vi "read_lia.vi"(5 "Samples per step":i32, 6 "Reference Source (0: Internal)":i32(ring)=1 items=["Internal", "External", "Dual", "Chop"], 7 "error in (no error)":errorcluster, 8 "Single Lock-in Parameter 2 (0: X output)":i32(ring)=3 items=["X output", "Y output", "R output", "Theta output", "Aux In 1", "Aux In 2", "Aux In 3", "Aux In 4", "Aux Out 1", "Aux Out 2", "Xnoise", "Ynoise", "Reference Phase", "Sine Out Amplitude", "DC Level", "Int. Ref. Frequency", "Ext. Ref. Frequency"], 9 "Single Lock-in Parameter (0: X output)":u16(ring)=2 items=["X output", "Y output", "R output", "Theta output", "Aux In 1", "Aux In 2", "Aux In 3", "Aux In 4", "Aux Out 1", "Aux Out 2", "Xnoise", "Ynoise", "Reference Phase", "Sine Out Amplitude", "DC Level", "Int. Ref. Frequency", "Ext. Ref. Frequency"], 10 "VISA resource name":refnum<visa-resource-name>="SR865") -> (0 "error out":errorcluster, 1 "Output 2":dbl, 2 "Output 1":dbl, 3 "VISA resource name out":refnum<visa-resource-name>)   [LabVIEW 2018]
uses:
  <instrlib>/Stanford Research SR865/Stanford Research SR865.lvlib
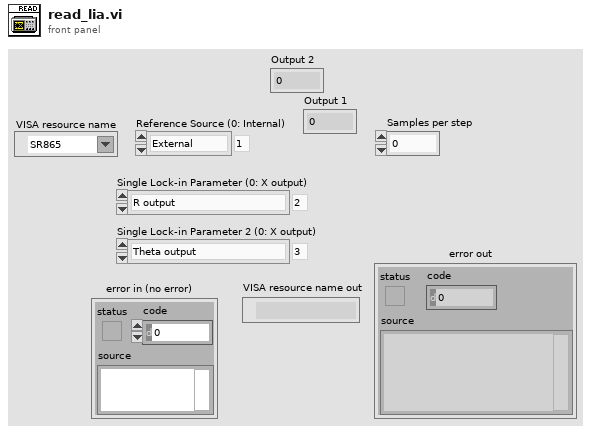
[diagram p1: front panel]
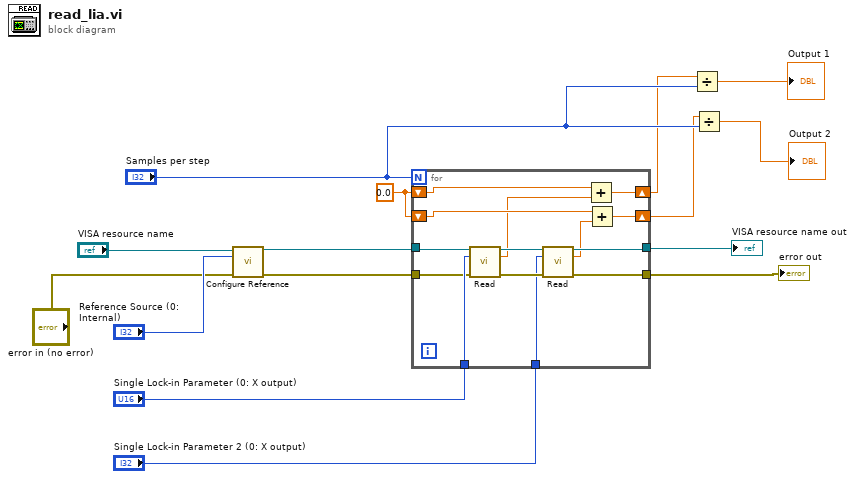
[diagram p0: block diagram]
diagram:
  w6 = 0.0
  n1 = call <instrlib>:"Configure Reference.vi"("VISA resource name"="VISA resource name", "Reference Source (0: Internal)"="Reference Source (0: Internal)", "error in (no error)"="error in (no error)") -> ("VISA resource name out"=w11:refnum<visa-resource-name>, "error out"=w9:errorcluster)  [unwired: 11 in]
  n2 = for {
    N: "Samples per step" -> [_]
    tunnel: "Single Lock-in Parameter 2 (0: X output)" -> [w27]
    tunnel: w11 -> [w26]
    tunnel: "Single Lock-in Parameter (0: X output)" -> [w25]
    tunnel: w9 -> [w24]
    tunnel: [w23] -> w8
    tunnel: [w22] -> w7
    shift-right: [w21] -> w3
    shift-left: w6 -> [w18]
    shift-right: [w20] -> w4
    shift-left: w6 -> [w19]
    n3 = call <instrlib>:"Read.vi"("VISA resource name"=w26, "Single Lock-in Parameter (0: X output)"=w25, "error in (no error)"=w24) -> ("VISA resource name out"=w28:refnum<visa-resource-name>, "Single Lock-in Value"=w17:dbl, "error out"=w29:errorcluster)  [unwired: 8 in, 2 out]
    n4 = call <instrlib>:"Read.vi"("VISA resource name"=w28, "Single Lock-in Parameter (0: X output)"=w27, "error in (no error)"=w29) -> ("VISA resource name out"=w23:refnum<visa-resource-name>, "Single Lock-in Value"=w16:dbl, "error out"=w22:errorcluster)  [unwired: 8 in, 2 out]
    n5 = Add(x=w19, y=w17) -> (x+y=w20:dbl)
    n6 = Add(x=w18, y=w16) -> (x+y=w21:dbl)
  }
  "VISA resource name out" <- w8
  "error out" <- w7
  n7 = Divide(x=w4, y="Samples per step") -> (x/y=→"Output 1":dbl)
  n8 = Divide(x=w3, y="Samples per step") -> (x/y=→"Output 2":dbl)
